vi "io_read_OPC.vi"(6 "Block Logging (F)":bool, 8 "error in":errorcluster caption="error in (no error)", 11 "VISA resource name":refnum<visa-resource-name>) -> (0 "error out":errorcluster, 2 "OPC returned":i32 format="%.0x", 3 "VISA resource name out":refnum<visa-resource-name>)   [LabVIEW 2022 SP3, in "hmp4000_rsidr_core.lvlib"]
uses:
  hmp4000_rsidr_core.lvlib
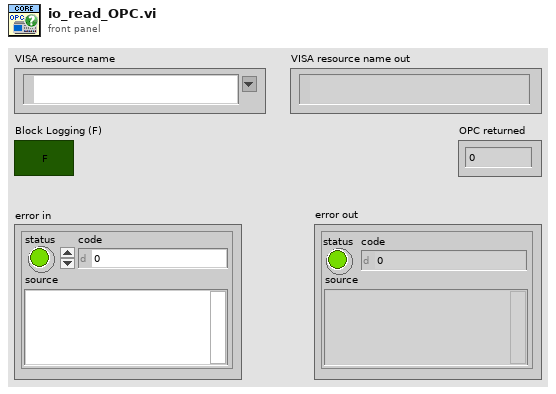
[diagram p1: front panel]
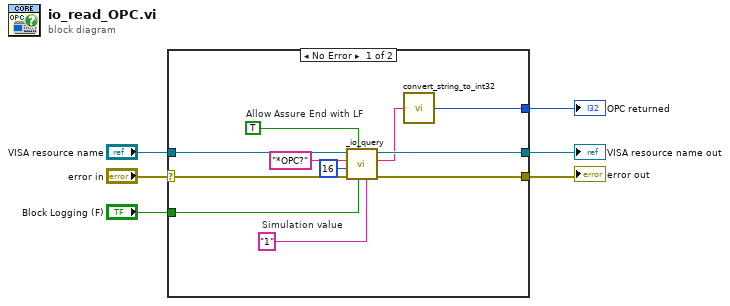
[diagram p0: block diagram]
diagram:
  n1 = case shown="No Error" "error in" {
    selector: "error in" -> [w14 w19]
    tunnel: [w17 w19] -> w6
    tunnel: "VISA resource name" -> [w15 w18]
    tunnel: [w10 _] -> w5
    tunnel: [w16 w18] -> w2
    tunnel: "Block Logging (F)" -> [w9 _]
    frame No Error {
      w7 = TRUE  # Allow Assure End with LF
      w8 = "1"  # Simulation value
      n2 = call "_io_query.vi"("Simulation read buffer (\"Simulation\")"=w8, "Block Logging (F)"=w9, "Allow Assure End with LF"=w7, "error in"=w14, "Max bytes to read (2048)"=u32 16 ("Bytes to read (1024)"), "Write buffer"="*OPC?" ("write buffer"), "VISA resource name"=w15) -> ("error out"=w17:errorcluster, "Read buffer"=w11:string, "VISA resource name out"=w16:refnum<visa-resource-name>)  [unwired: 1 in, 1 out]
      n3 = call "convert_string_to_int32.vi"("String in"=w11) -> ("int32 value out"=w10:i32)  [unwired: 4 in]
    }
    frame Error {
    }
  }
  "VISA resource name out" <- w2
  "error out" <- w6
  "OPC returned" <- w5
